vi "ke37xx Scan List.vi"(0 "VISA Resource Name":refnum<visa-resource-name>, 1 "Channel List":string, 5 "Action (0: Create)":T1(ring), 7 "Configuration":string, 11 "error in (no error)":errorcluster, 12 "Bytes To Read (1024)":u32=1024) -> (4 "VISA Resource Name Out":refnum<visa-resource-name>, 8 "Scan List":string, 15 "error out":errorcluster)   [LabVIEW 2009, in "Keithley 3700 Series.lvlib"]
doc: "This VI allows you to create, append, or query a scan list, or add multiple channels to a scan step."
uses:
  <instrlib>/Keithley 3706/Keithley 3700 Series.lvlib
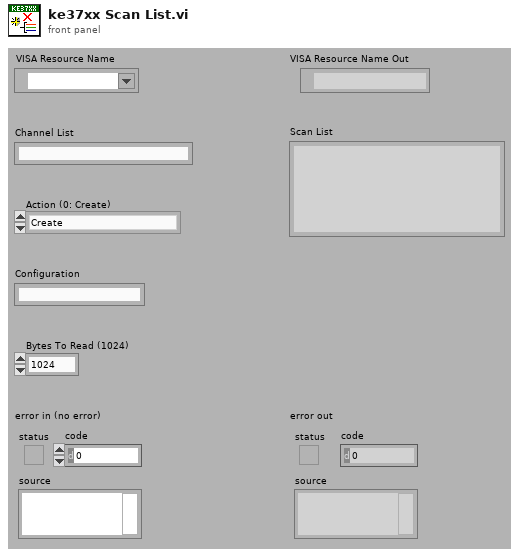
[diagram p1: front panel]
types:
  T1 = enum16{"Create", "Append", "Query", "Append Multi Channel Step"}
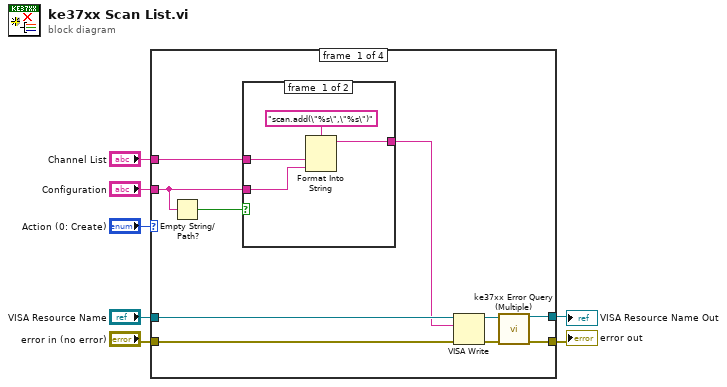
[diagram p0: block diagram]
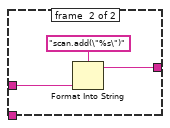
[diagram p2: hidden frame]
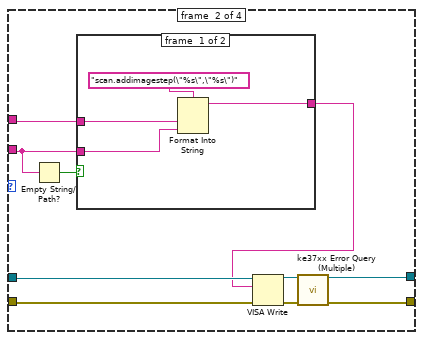
[diagram p3: hidden frame]
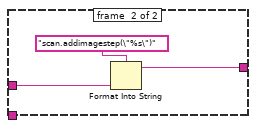
[diagram p4: hidden frame]
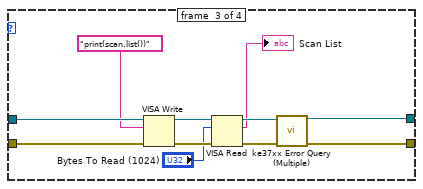
[diagram p5: hidden frame]
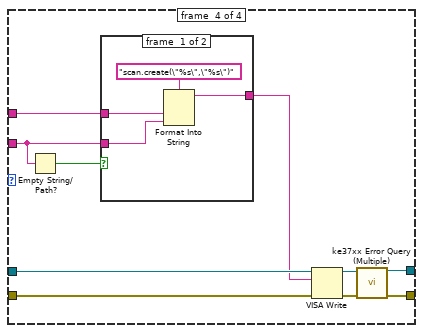
[diagram p6: hidden frame]
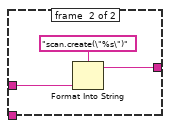
[diagram p7: hidden frame]
diagram:
  n1 = case shown="\"Create\", Default" "Action (0: Create)" {
    tunnel: [w17 w31 w52 w62] -> w7
    tunnel: [w16 w30 w51 w61] -> w6
    tunnel: "VISA Resource Name" -> [w15 w27 w50 w60]
    tunnel: "error in (no error)" -> [w14 w26 w49 w59]
    tunnel: "Configuration" -> [w9 w32 _ w54]
    tunnel: "Channel List" -> [w10 w34 _ w55]
    frame #0 {
      n2 = Empty String/Path?(string/path=w9) -> (empty?=w11:bool)
      n3 = case shown="False" w11 {
        tunnel: w10 -> [w20 w23]
        tunnel: w9 -> [w19 _]
        tunnel: [w18 w22] -> w8
        frame #0 {
          n4 = Format Into String(format string="scan.add(\"%s\",\"%s\")", w20, w19) -> (resulting string=w18:string)  [unwired: 2 in, 1 out]
        }
        frame #1 {
          n5 = Format Into String(format string="scan.add(\"%s\")", w23) -> (resulting string=w22:string)  [unwired: 2 in, 1 out]
        }
      }
      n6 = VISA Write(VISA resource name=w15, write buffer=w8, error in (no error)=w14) -> (VISA resource name out=w13:refnum<visa-resource-name>, error out=w12:errorcluster)  [unwired: 1 out]
      n7 = call <instrlib>:"ke37xx Error Query (Multiple).vi"("VISA resource name"=w13, "error in (no error)"=w12) -> ("VISA resource name out"=w17:refnum<visa-resource-name>, "error out"=w16:errorcluster)  [unwired: 12 out]
    }
    frame #1 {
      n8 = Empty String/Path?(string/path=w32) -> (empty?=w33:bool)
      n9 = case shown="True" w33 {
        tunnel: w34 -> [w37 w40]
        tunnel: w32 -> [w36 _]
        tunnel: [w35 w39] -> w25
        frame #0 {
          n10 = Format Into String(format string="scan.addimagestep(\"%s\",\"%s\")", w37, w36) -> (resulting string=w35:string)  [unwired: 2 in, 1 out]
        }
        frame #1 {
          n11 = Format Into String(format string="scan.addimagestep(\"%s\")", w40) -> (resulting string=w39:string)  [unwired: 2 in, 1 out]
        }
      }
      n12 = VISA Write(VISA resource name=w27, write buffer=w25, error in (no error)=w26) -> (VISA resource name out=w28:refnum<visa-resource-name>, error out=w29:errorcluster)  [unwired: 1 out]
      n13 = call <instrlib>:"ke37xx Error Query (Multiple).vi"("VISA resource name"=w28, "error in (no error)"=w29) -> ("VISA resource name out"=w31:refnum<visa-resource-name>, "error out"=w30:errorcluster)  [unwired: 12 out]
    }
    frame #2 {
      n14 = VISA Write(VISA resource name=w50, write buffer="print(scan.list())", error in (no error)=w49) -> (VISA resource name out=w47:refnum<visa-resource-name>, error out=w48:errorcluster)  [unwired: 1 out]
      n15 = VISA Read(VISA resource name=w47, byte count="Bytes To Read (1024)", error in (no error)=w48) -> (VISA resource name out=w46:refnum<visa-resource-name>, read buffer=→"Scan List":string, error out=w45:errorcluster)  [unwired: 1 out]
      n16 = call <instrlib>:"ke37xx Error Query (Multiple).vi"("VISA resource name"=w46, "error in (no error)"=w45) -> ("VISA resource name out"=w52:refnum<visa-resource-name>, "error out"=w51:errorcluster)  [unwired: 12 out]
    }
    frame #3 {
      n17 = Empty String/Path?(string/path=w54) -> (empty?=w56:bool)
      n18 = case shown="False" w56 {
        tunnel: w55 -> [w65 w68]
        tunnel: w54 -> [w64 _]
        tunnel: [w63 w67] -> w53
        frame #0 {
          n19 = Format Into String(format string="scan.create(\"%s\",\"%s\")", w65, w64) -> (resulting string=w63:string)  [unwired: 2 in, 1 out]
        }
        frame #1 {
          n20 = Format Into String(format string="scan.create(\"%s\")", w68) -> (resulting string=w67:string)  [unwired: 2 in, 1 out]
        }
      }
      n21 = VISA Write(VISA resource name=w60, write buffer=w53, error in (no error)=w59) -> (VISA resource name out=w58:refnum<visa-resource-name>, error out=w57:errorcluster)  [unwired: 1 out]
      n22 = call <instrlib>:"ke37xx Error Query (Multiple).vi"("VISA resource name"=w58, "error in (no error)"=w57) -> ("VISA resource name out"=w62:refnum<visa-resource-name>, "error out"=w61:errorcluster)  [unwired: 12 out]
    }
  }
  "VISA Resource Name Out" <- w7
  "error out" <- w6
